vi "Zmien pozycje liniowo.vi"(8 "error in (no error)":errorcluster, 11 "Swiat in":refnum<class "Swiat.lvclass">) -> (0 "error out":errorcluster, 3 "Swiat out":refnum<class "Swiat.lvclass">)   [LabVIEW 2014, in "Swiat.lvclass"]
uses:
  Swiat.lvclass
  Swiat.lvclass/Swiat.ctl
  Boid/Boid.lvclass/Boid.ctl
  Boid/Boid.lvclass
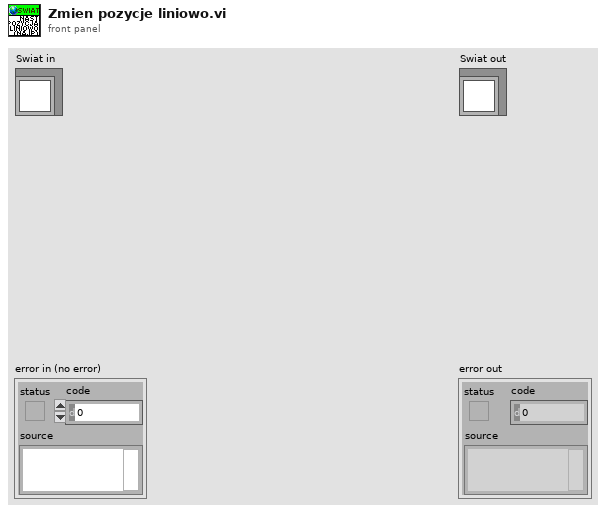
[diagram p1: front panel]
types:
  T1 = typedef "LVBoundsTypeDef.ctl" = cluster{"Width":u32, "Height":u32}
  T2 = typedef "Position.ctl" = cluster{"x":i16, "y":i16}
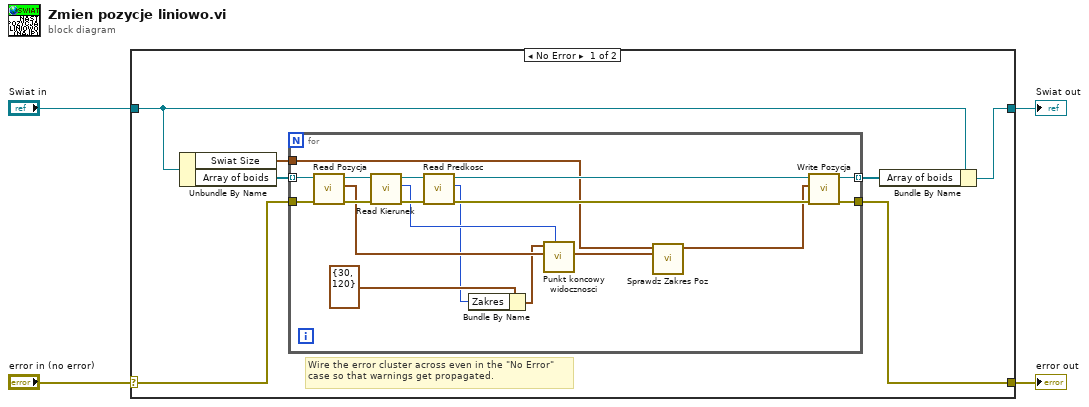
[diagram p0: block diagram]
diagram:
  n1 = case shown="No Error" "error in (no error)" {
    selector: "error in (no error)" -> [w7 w30]
    tunnel: [w6 w30] -> w1
    tunnel: [w10 w31] -> w2
    tunnel: "Swiat in" -> [w11 w31]
    frame No Error {
      # "Wire the error cluster across even in the \"No Error\"\ncase so that warnings get propagated."
      n2 = Unbundle By Name(w11) -> ("Swiat Size"=w5:T1, "Array of boids"=w9:refnum<class "Boid.lvclass">[])
      n3 = for {
        tunnel: w9 -> [w29] mode=indexing
        tunnel: w7 -> [w27]
        tunnel: [w21] -> w8 mode=indexing
        tunnel: [w20] -> w6
        tunnel: w5 -> [w12]
        n4 = call "Read Pozycja.vi"("error in (no error)"=w27, "Boid in"=w29) -> ("error out"=w26:errorcluster, "Position"=w19:T2, "Boid out"=w28:refnum<class "Boid.lvclass">)  [unwired: 7 in]
        n5 = call "Read Kierunek.vi"("error in (no error)"=w26, "Boid in"=w28) -> ("error out"=w25:errorcluster, "Kierunek"=w18:i16, "Boid out"=w24:refnum<class "Boid.lvclass">)  [unwired: 7 in]
        n6 = call "Read Predkosc.vi"("error in (no error)"=w25, "Boid in"=w24) -> ("error out"=w22:errorcluster, "Predkosc"=w15:i16, "Boid out"=w23:refnum<class "Boid.lvclass">)  [unwired: 7 in]
        n7 = Bundle By Name(cluster=cluster{"Zakres":i16, "Kat":i16} {"Zakres"=30, "Kat"=120} ("Percepcja"), "Zakres"=w15) -> (w16:cluster{"Zakres":i16, "Kat":i16})
        n8 = call "Punkt koncowy widocznosci.vi"("Kierunek"=w18, "Start Pos"=w19, "Percepcja"=w16) -> ("Final Pos"=w14:T2)  [unwired: 7 in, 1 out]
        n9 = call "Sprawdz Zakres Poz.vi"("Pos in"=w14, "Swiat Size"=w12) -> ("Pos out"=w13:T2)  [unwired: 8 in, 1 out]
        n10 = call "Write Pozycja.vi"("error in (no error)"=w22, "Position"=w13, "Boid in"=w23) -> ("error out"=w20:errorcluster, "Boid out"=w21:refnum<class "Boid.lvclass">)  [unwired: 7 in]
      }
      n11 = Bundle By Name(cluster=w11, "Array of boids"=w8) -> (w10:refnum<class "Swiat.lvclass">)
    }
    frame Error {
    }
  }
  "error out" <- w1
  "Swiat out" <- w2
